vi "kinectRead [BodyFrame].vi"(8 "error in (no error)":errorcluster, 9 "Timeout (ms)":i32=5000, 11 "KinectSensor References in":T2) -> (0 "error out":errorcluster, 2 "Body Data":T1[](array[typedef]) {"LeanTrackingState" items=["NotTracked", "Inferred", "Tracked"]; "HandRightState" items=["Unknown", "NotTracked", "Open", "Closed", "Lasso"]; "HandRightConfidence" items=["Low", "High"]; "HandLeftState" items=["Unknown", "NotTracked", "Open", "Closed", "Lasso"]; "HandLeftConfidence" items=["Low", "High"]; "ClippedEdges" items=["None"=0, "Right"=1, "Left"=2, "Top"=4, "Bottom"=8]}, 3 "KinectSensor References out":T2)   [LabVIEW 2014, in "LVH-KinectOne.lvlib"]
uses:
  LVH-KinectOne.lvlib
  Type Defs/KinectSensor References.ctl
  Microsoft.Kinect
  C:/github/labviewhacker/LVH-KinectOne/LabVIEW/vi.lib/LabVIEW Hacker/KinectOne/Private/Libs/BodyFrameDataInterface.dll
  Libs/BodyFrameDataInterface.dll
  Type Defs/BodyData.ctl
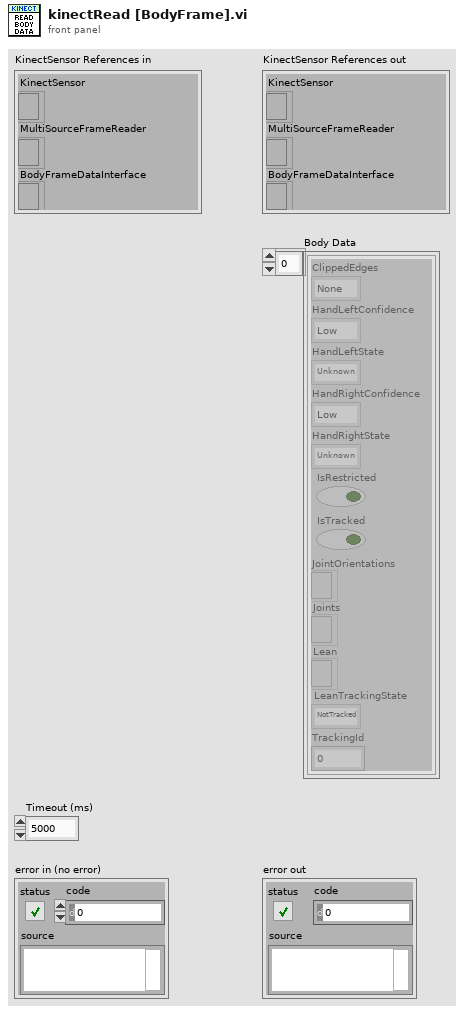
[diagram p1: front panel]
types:
  T1 = typedef "LVH-KinectOne.lvlib/BodyData.ctl" = cluster{"ClippedEdges":i32, "HandLeftConfidence":i32, "HandLeftState":i32, "HandRightConfidence":i32, "HandRightState":i32, "IsRestricted":bool, "IsTracked":bool, "JointOrientations":refnum<k24>, "Joints":refnum<k24>, "Lean":refnum<k24>, "LeanTrackingState":i32, "TrackingId":u64}
  T2 = typedef "LVH-KinectOne.lvlib/KinectSensor References.ctl" = cluster{"KinectSensor":refnum<k24>, "MultiSourceFrameReader":refnum<k24>, "BodyFrameDataInterface":refnum<k24>}
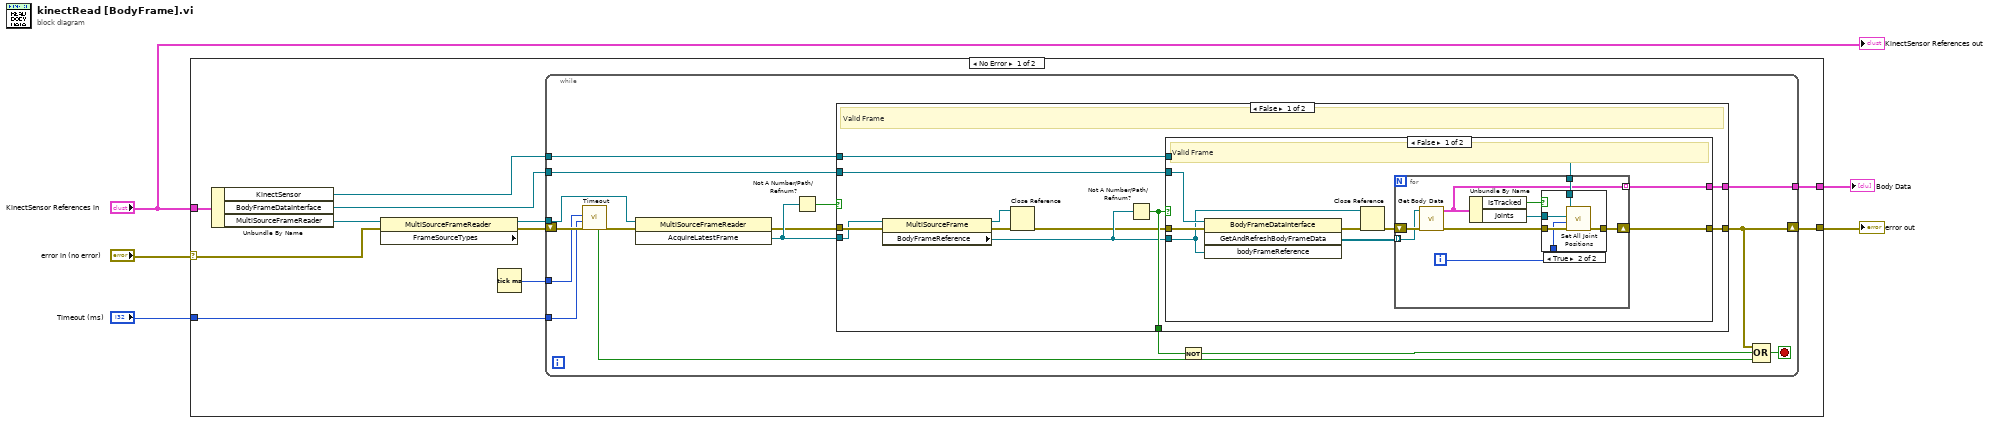
[diagram p0: block diagram]
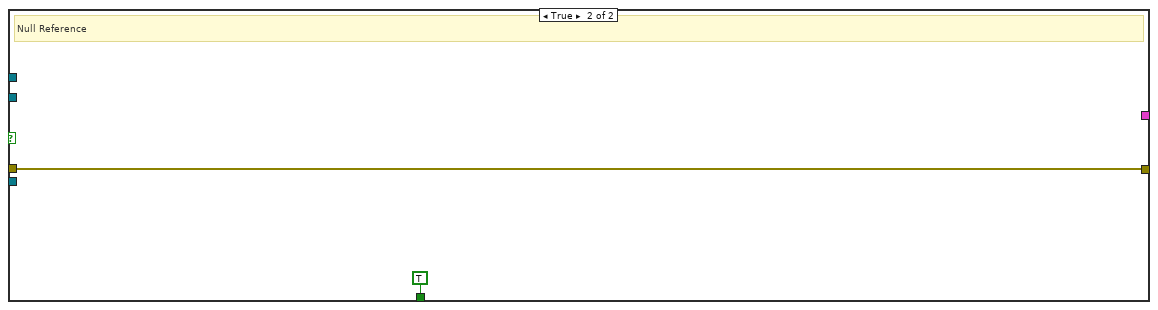
[diagram p4: hidden frame]
diagram:
  n1 = case shown="No Error" "error in (no error)" {
    selector: "error in (no error)" -> [w7 w71]
    tunnel: "KinectSensor References in" -> [w13 _]
    tunnel: [w12 w71] -> w4
    tunnel: [w11 _] -> w3
    tunnel: "Timeout (ms)" -> [w8 _]
    frame No Error {
      n2 = Unbundle By Name(w13) -> ("KinectSensor"=w6:refnum<k24>, "BodyFrameDataInterface"=w10:refnum<k24>, "MultiSourceFrameReader"=w14:refnum<k24>)
      n3 = property class="MultiSourceFrameReader" props=["FrameSourceTypes"](reference=w14, error in=w7) -> (reference out=w16:refnum<k24>, error out=w15:errorcluster)  [unwired: 1 out]
      n4 = Tick Count (ms)() -> (millisecond timer value=w9:u32)
      n5 = while {
        tunnel: w16 -> [w27]
        shift-right: [w22] -> w12
        shift-left: w15 -> [w26]
        tunnel: [w29] -> w11
        tunnel: w10 -> [w28]
        tunnel: w9 -> [w24]
        tunnel: w8 -> [w23]
        tunnel: w6 -> [w17]
        stop <- w21 stop-if-true
        n6 = call "Timeout.vi"("error in (no error)"=w26, "Timeout (ms)"=w23, "Start Time"=w24) -> ("error out"=w25:errorcluster, "Timeout?"=w18:bool)  [unwired: 7 in]
        n7 = invoke class="MultiSourceFrameReader" method="AcquireLatestFrame"(reference=w27, error in=w25) -> (error out=w31:errorcluster, "AcquireLatestFrame"=w32:refnum<k24>)  [unwired: 1 in, 1 out]
        n8 = Not A Number/Path/Refnum?(number/path/refnum=w32) -> (NaN/Path/Refnum?=w30:bool)
        n9 = case shown="False" w30 {
          tunnel: w31 -> [w43 w69]
          tunnel: w32 -> [w40 _]
          tunnel: [w42 w69] -> w22
          tunnel: [w41 TRUE] -> w20
          tunnel: w28 -> [w39 _]
          tunnel: [w38 _] -> w29
          tunnel: w17 -> [w36 _]
          frame False {
            # "Valid Frame"
            n10 = property class="MultiSourceFrame"(reference=w40, error in=w43) -> (reference out=w34:refnum<k24>, error out=w35:errorcluster, "BodyFrameReference"=w37:refnum<k24>)
            n11 = Close Reference(reference=w34, error in (no error)=w35) -> (error out=w33:errorcluster)
            n12 = Not A Number/Path/Refnum?(number/path/refnum=w37) -> (NaN/Path/Refnum?=w41:bool)
            n13 = case shown="False" w41 {
              tunnel: [w48 w68] -> w42
              tunnel: w39 -> [w51 _]
              tunnel: [w50 _] -> w38
              tunnel: w33 -> [w49 w68]
              tunnel: w37 -> [w44 _]
              tunnel: w36 -> [w47 _]
              frame False {
                # "Valid Frame"
                n14 = invoke class="BodyFrameDataInterface" method="GetAndRefreshBodyFrameData"(reference=w51, error in=w49, "bodyFrameReference"=w44) -> (error out=w46:errorcluster, "GetAndRefreshBodyFrameData"=w52:refnum<k24>[])  [unwired: 1 in, 2 out]
                n15 = Close Reference(reference=w44, error in (no error)=w46) -> (error out=w45:errorcluster)
                n16 = for {
                  tunnel: w52 -> [w60] mode=indexing
                  shift-right: [w59] -> w48
                  shift-left: w45 -> [w61]
                  tunnel: [w54] -> w50 mode=indexing
                  tunnel: w47 -> [w55]
                  i -> [w57]
                  n17 = call "Get Body Data.vi"("error in (no error)"=w61, "Body Reference"=w60) -> ("error out"=w58:errorcluster, "BodyData"=w54:T1)  [unwired: 8 in]
                  n18 = Unbundle By Name(w54) -> ("IsTracked"=w53:bool, "Joints"=w56:refnum<k24>)
                  n19 = case shown="True" w53 {
                    tunnel: [w62 w67] -> w59
                    tunnel: w58 -> [w62 w66]
                    tunnel: w57 -> [_ w65]
                    tunnel: w56 -> [_ w64]
                    tunnel: w55 -> [_ w63]
                    frame False {
                    }
                    frame True {
                      n20 = call "Set All Joint Positions.vi"("error in (no error)"=w66, "Body Index"=w65, "Joints"=w64, "KinectSensor Reference"=w63) -> ("error out"=w67:errorcluster)  [unwired: 7 in]
                    }
                  }
                }
              }
              frame True {
                # "Null Reference"
              }
            }
          }
          frame True {
            # "Null Reference"
          }
        }
        n21 = Not(x=w20) -> (.not. x?=w19:bool)
        n22 = Compound Arithmetic op=OR(w22, w19, w18) -> (w21:bool)
      }
    }
    frame Error {
    }
  }
  "error out" <- w4
  "Body Data" <- w3
  "KinectSensor References out" <- "KinectSensor References in"
